vi "GetLoggerRef.vi"(8 "error in (no error)":errorcluster caption="错误输入（无错误）", 10 "LoggerSavePath":path) -> (0 "error out":errorcluster, 2 "refnum":refnum<file>)   [LabVIEW 2019, in "Logger.lvclass"]
uses:
  <userlib>/Logger/Logger.lvclass
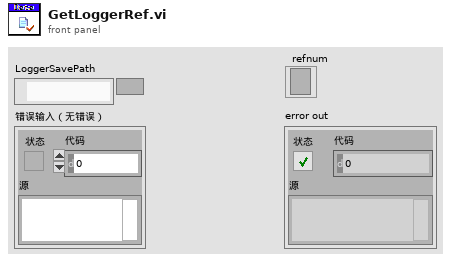
[diagram p1: front panel]
types:
  T1 = enum16{"open", "replace", "create", "open or create", "replace or create", "replace or create with confirmation"}
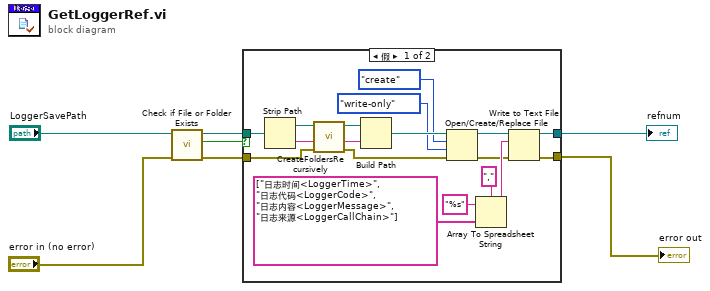
[diagram p0: block diagram]
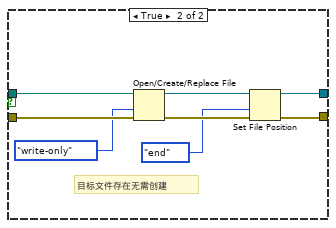
[diagram p2: hidden frame]
diagram:
  n1 = call <vilib>:"Check if File or Folder Exists.vi"("error in (no error)"="error in (no error)", "path"="LoggerSavePath") -> ("error out"=w3:errorcluster, "file or folder exists?"=w5:bool, "dup path"=w4:path)  [unwired: 7 in]
  n2 = case shown="假" w5 {
    tunnel: w4 -> [w18 w32]
    tunnel: w3 -> [w14 w29]
    tunnel: [w20 w26] -> w2
    tunnel: [w21 w27] -> w1
    frame False {
      n3 = Strip Path(path=w18) -> (stripped path=w17:path, name=w15:string)
      n4 = call <userlib>:"CreateFoldersRecursively.vi"("error in (no error)"=w14, "directory"=w17) -> ("error out"=w11:errorcluster, "directory copy"=w16:path)  [unwired: 7 in, 1 out]
      n5 = Build Path(base path=w16, name or relative path=w15) -> (appended path=w13:path)
      n6 = Open/Create/Replace File(file path (use dialog)=w13, error in=w11, operation (0:open)=T1."create" ("操作(0:open)"), access (0:read/write)=enum16{"read/write", "read-only", "write-only"}."write-only" ("权限(0:read/write)")) -> (refnum out=w9:refnum<file>, error out=w8:errorcluster)  [unwired: 2 in, 1 out]
      n7 = Array To Spreadsheet String(delimiter (Tab)="," ("分隔符(Tab)"), array=string[] ["日志时间<LoggerTime>", "日志代码<LoggerCode>", "日志内容<LoggerMessage>", "日志来源<LoggerCallChain>"], 3:"%s" ("格式字符串")) -> (spreadsheet string=w22:string)
      n8 = Write to Text File(file (use dialog)=w9, text=w22, error in=w8) -> (refnum out=w21:refnum<file>, error out=w20:errorcluster)  [unwired: 1 in, 1 out]
    }
    frame True {
      # "目标文件存在无需创建"
      n9 = Open/Create/Replace File(file path (use dialog)=w32, error in=w29, access (0:read/write)=enum16{"read/write", "read-only", "write-only"}."write-only" ("权限(0:read/write)")) -> (refnum out=w30:refnum<file>, error out=w31:errorcluster)  [unwired: 3 in, 1 out]
      n10 = Set File Position(refnum=w30, from (0:start)=enum16{"start", "end", "current"}."end" ("自（0:起始）"), error in=w31) -> (refnum out=w27:refnum<file>, error out=w26:errorcluster)  [unwired: 1 in]
    }
  }
  "error out" <- w2
  "refnum" <- w1
